vi "SetClassQueue.vi"(8 "ErrorIn(No Error)":errorcluster caption="entrée d'erreur (pas d'erreur)", 10 "Menu déroulant":T1 items=["UpdateClassData", "UpdateMainClass"], 11 "DefaultDev.lvclass":refnum<class "ThorPM100A.lvclass">) -> (0 "sortie d'erreur":errorcluster, 3 "DefaultDev.lvclass Out":refnum<class "ThorPM100A.lvclass">)   [LabVIEW 2019, in "ThorPM100A.lvclass"]
uses:
  ThorPM100A.lvclass
  BaseDevice/ClassQueueMess.ctl
  BaseDevice/BaseDevice.lvclass
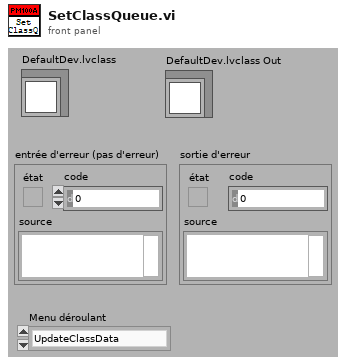
[diagram p1: front panel]
types:
  T1 = typedef "ClassQueueMess.ctl" = u16
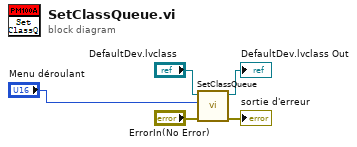
[diagram p0: block diagram]
diagram:
  n1 = call-parent "SetClassQueue.vi"("ErrorIn(No Error)"="ErrorIn(No Error)", "Menu déroulant"="Menu déroulant", "BaseDevice.lvclass"="DefaultDev.lvclass") -> ("sortie d'erreur"=→"sortie d'erreur":errorcluster, "BaseDevice.lvclass Out"=→"DefaultDev.lvclass Out":refnum<class "ThorPM100A.lvclass">)  [unwired: 7 in]
